vi "主程序.vi"() -> ()   [LabVIEW 2016]
panel:
  out "数值":dbl
  in  "y":dbl
  in  "x":dbl
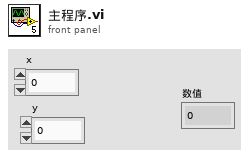
[diagram p1: front panel]
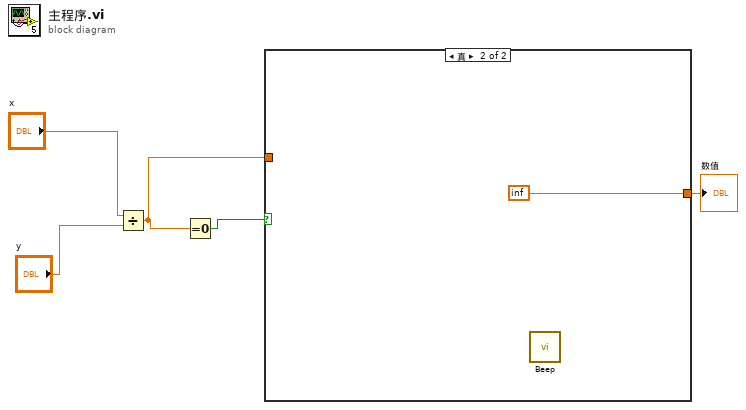
[diagram p0: block diagram]
diagram:
  n1 = Divide(x="x", y="y") -> (x/y=w1:dbl)
  n2 = Equal To 0?(x=w1) -> (x = 0?=w3:bool)
  n3 = case shown="真" w3 {
    tunnel: [w6 inf] -> w2
    tunnel: w1 -> [w6 _]
    frame False {
    }
    frame True {
      n4 = call <vilib>:"Beep.vi"() -> ()  [unwired: 12 in]
    }
  }
  "数值" <- w2
